vi "component orientation check.vi"(8 "error in":errorcluster, 10 "input cluster":T1, 11 "Gantry In":refnum<k24>) -> (0 "error out":errorcluster, 1 "Wrong Orientation?":bool, 2 "output cluster":T1, 3 "Gantry Out":refnum<k24>)   [LabVIEW 2021, in "Component Tray.lvclass"]
uses:
  Component Tray.lvclass
  Find Component.ctl
  Controller/Camera/Machine Vision.ctl
  C:/Program Files (x86)/Aerotech/A3200/LabVIEW/2010/Bin/Aerotech.A3200.dll
  Program Files (x86)/Aerotech/A3200/LabVIEW/2010/Bin/Aerotech.A3200.dll
  Component Tray.lvclass/Component Tray.ctl
  Controller/Motion/A3200/A3200.lvclass
  Controller/Camera/Camera.lvclass
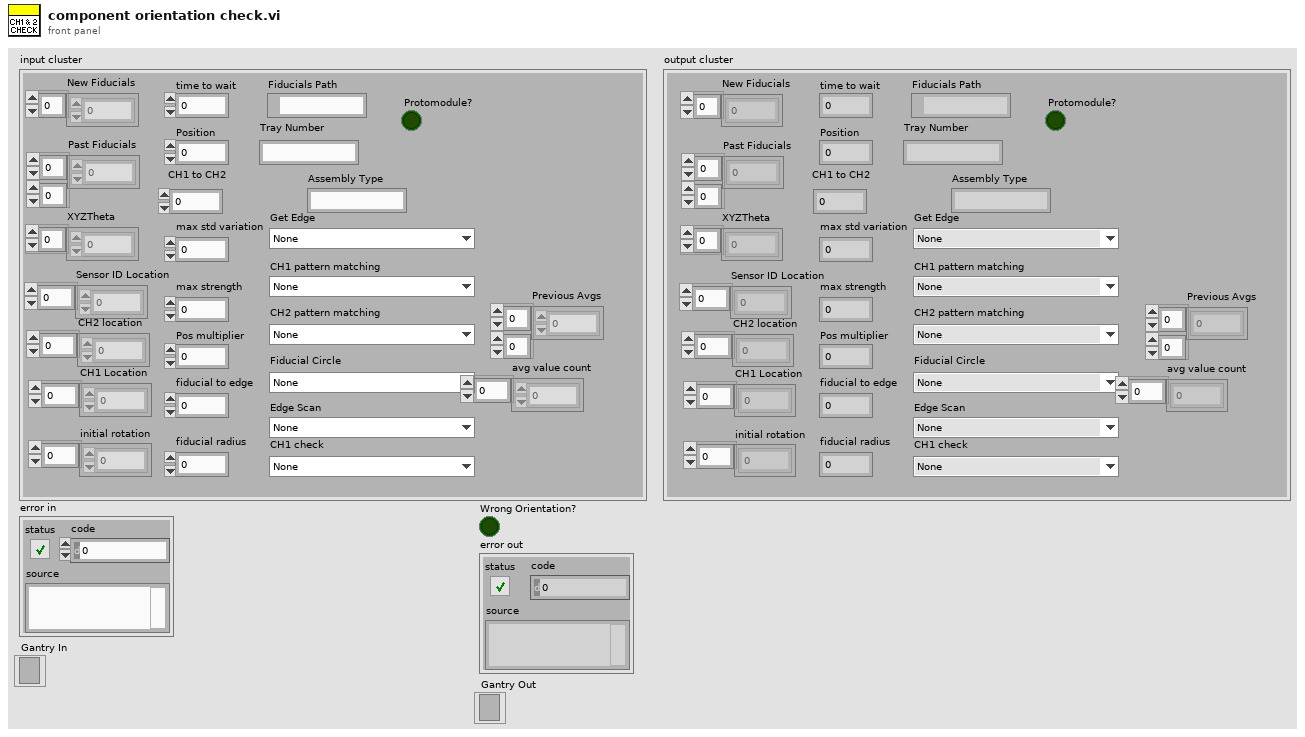
[diagram p1: front panel]
types:
  T1 = typedef "Component Tray.lvclass/Find Component.ctl" = cluster{"New Fiducials":dbl[], "Past Fiducials":dbl[][], "XYZTheta":dbl[], "Fiducials Path":path, "Position":i32, "CH1 Location":dbl[], "Sensor ID Location":dbl[], "initial rotation":dbl[], "CH2 location":dbl[], "max std variation":dbl, "max strength":dbl, "CH2 pattern matching":T2, "Fiducial Circle":T2, "Get Edge":T2, "Pos multiplier":dbl, "time to wait":u32, "fiducial to edge":dbl, "Protomodule?":bool, "Assembly Type":string, "CH1 to CH2":dbl, "Tray Number":string, "fiducial radius":dbl, "4 fiducials?":bool, "CH1 check":T2, "Edge Scan":T2, "CH1 pattern matching":T2, "Sensor Thickness":dbl, "Previous Avgs":dbl[][], "avg value count":dbl[]}
  T2 = typedef "Camera.lvclass/Machine Vision.ctl" = enum16{"None", "Assembly Tray Circle", "Assembly Tray Fiducial", "Partial Hexaboard", "sensor edge init", "HB edge init", "sensor edge pos1", "sensor edge pos2", "HB edge pos1", "HB edge pos2", "Sensor CH1-2", "HB CH1", "HB CH2", "V3 Sensor Circle", "Hexaboard Circle", "sensor CH1 check", "HB CH1 check ", "sensor ID"}
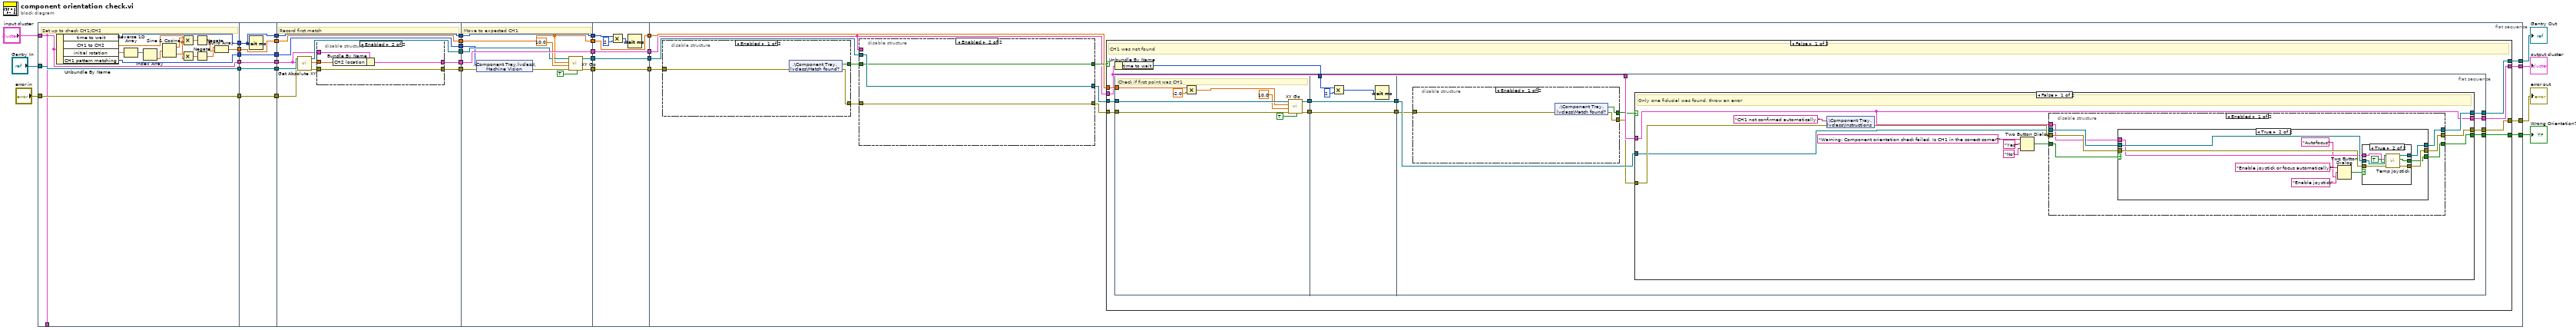
[diagram p0: block diagram]
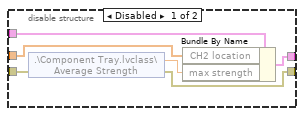
[diagram p2: hidden frame]
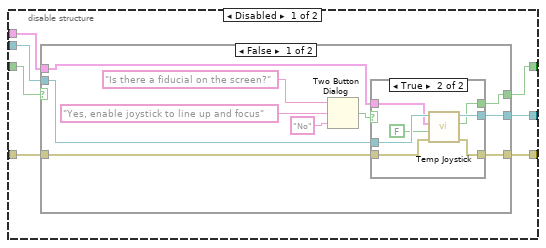
[diagram p3: hidden frame]
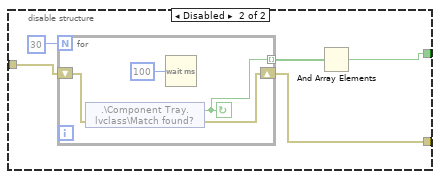
[diagram p6: hidden frame]
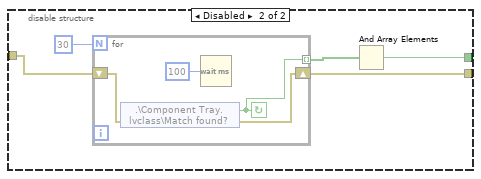
[diagram p7: hidden frame]
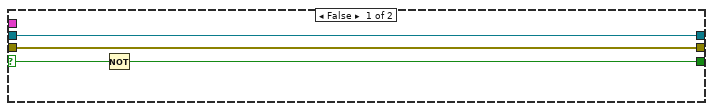
[diagram p8: hidden frame]
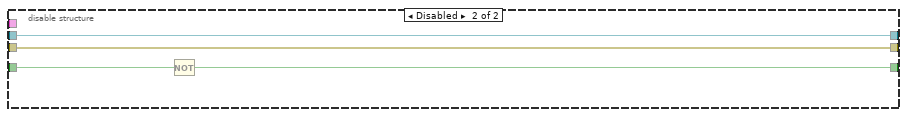
[diagram p10: hidden frame]
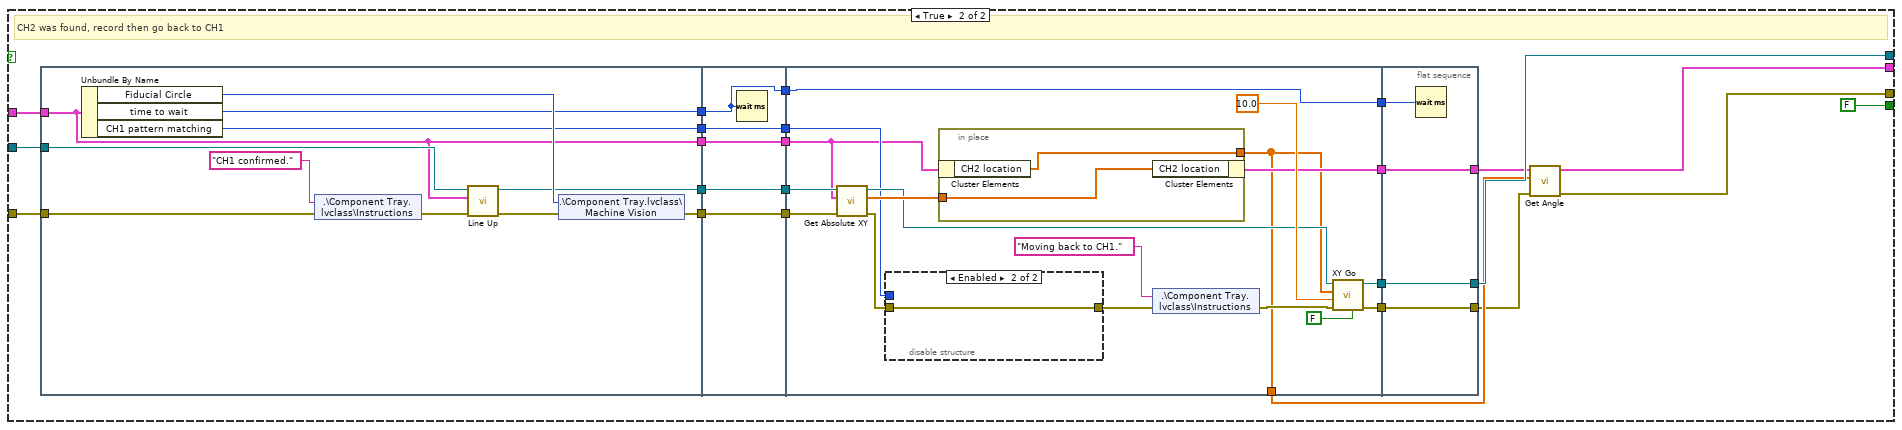
[diagram p11: hidden frame]
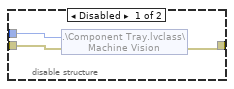
[diagram p12: hidden frame]
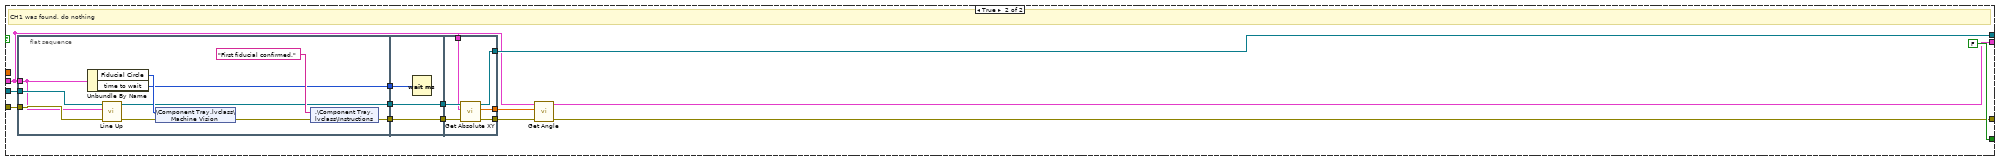
[diagram p13: hidden frame]
diagram:
  n1 = flat-sequence {
    tunnel: [w41] -> w27
    tunnel: [w40] -> w26
    tunnel: [w35] -> w25
    tunnel: [w50] -> w24
    tunnel: [w43] -> w23
    tunnel: [w42] -> w22
    tunnel: "input cluster" -> [w35]
    tunnel: "error in" -> [w40]
    tunnel: "Gantry In" -> [w41]
    tunnel: [w35] -> _
    tunnel: w27 -> [w56]
    tunnel: [w56] -> w21
    tunnel: w26 -> [w55]
    tunnel: [w55] -> w20
    tunnel: w25 -> [w54]
    tunnel: [w54] -> w19
    tunnel: w24 -> [w53]
    tunnel: [w53] -> w18
    tunnel: w23 -> [w52]
    tunnel: [w52] -> w17
    tunnel: w22 -> [w51]
    tunnel: [w51] -> w16
    tunnel: w21 -> [w66]
    tunnel: w20 -> [w65]
    tunnel: w19 -> [w57]
    tunnel: w18 -> [w60]
    tunnel: w17 -> [w63]
    tunnel: [w64] -> w15
    tunnel: [w58] -> w14
    tunnel: [w63] -> w13
    tunnel: [w62] -> w12
    tunnel: [w61] -> w11
    tunnel: w16 -> [w61]
    tunnel: [w60] -> w10
    tunnel: w15 -> [w88]
    tunnel: w14 -> [w79]
    tunnel: w13 -> [w80]
    tunnel: w12 -> [w85]
    tunnel: w11 -> [w82]
    tunnel: [w83] -> w9
    tunnel: [w84] -> w8
    tunnel: [w88] -> w7
    tunnel: w10 -> [w81]
    tunnel: [w81] -> w6
    tunnel: [w80] -> w5
    tunnel: w9 -> [w95]
    tunnel: [w95] -> w4
    tunnel: w8 -> [w94]
    tunnel: [w94] -> w3
    tunnel: w7 -> [w93]
    tunnel: [w93] -> w2
    tunnel: w6 -> [w91]
    tunnel: w5 -> [w92]
    tunnel: [w92] -> w1
    tunnel: [w105] -> w28
    tunnel: [w107] -> w29
    tunnel: [w108] -> w34
    tunnel: w4 -> [w100]
    tunnel: w3 -> [w103]
    tunnel: w2 -> [w96]
    tunnel: w1 -> [w106]
    tunnel: [w104] -> w30
    frame #0 {
      # "Set up to check CH1/CH2"
      n2 = Unbundle By Name(w35) -> ("time to wait"=w50:u32, "CH1 to CH2"=w44:dbl, "initial rotation"=w45:dbl[], "CH1 pattern matching"=w42:T2)
      n3 = Reverse 1D Array(array=w45) -> (reversed array=w46:dbl[])
      n4 = Index Array(array=w46) -> (element=w49:dbl)  [unwired: 1 in]
      n5 = Sine & Cosine(0:w49) -> (1:w48:dbl, 2:w47:dbl)
      n6 = Multiply(x=w48, y=w44) -> (x*y=w39:dbl)
      n7 = Multiply(x=w47, y=w44) -> (x*y=w37:dbl)
      n8 = Negate(x=w39) -> (-x=w38:dbl)
      n9 = Negate(x=w37) -> (-x=w36:dbl)
      n10 = Build Array(w36, w38) -> (w43:dbl[])
    }
    frame #1 {
      n11 = Wait (ms)(milliseconds to wait=w53) -> ()  [unwired: 1 out]
    }
    frame #2 {
      # "Record first match"
      n12 = call "Get Absolute XY.vi"("error in (no error)"=w65, "Component"=w57, "Gantry In"=w66) -> ("error out"=w59:errorcluster, "Abs XY"=w67:dbl[], "Gantry Out"=w62:refnum<k24>)  [unwired: 6 in]
      n13 = disable-structure shown="Enabled" {
        disable-tunnel: w57 -> [w73 w76]
        disable-tunnel: w67 -> [w72 w77]
        disable-tunnel: [w71 w75] -> w64
        disable-tunnel: w59 -> [w69 w74]
        disable-tunnel: [w68 w74] -> w58
        frame Disabled {
          n14 = shared-variable ".\\Component Tray.lvclass\\Average Strength"(error in=w69) -> (w70:dbl, error out=w68:errorcluster)
          n15 = Bundle By Name(cluster=w73, "CH2 location"=w72, "max strength"=w70) -> (w71:T1)
        }
        frame Enabled {
          n16 = Bundle By Name(cluster=w76, "CH2 location"=w77) -> (w75:T1)
        }
      }
    }
    frame #3 {
      # "Move to expected CH1"
      n17 = shared-variable ".\\Component Tray.lvclass\\Machine Vision"(w82, error in=w79) -> (error out=w78:errorcluster)
      n18 = call "XY Go.vi"("Increment?"=TRUE, "error in (no error)"=w78, "Speed"=10.0, "XY In"=w80, "Gantry In"=w85) -> ("error out"=w84:errorcluster, "Gantry Out"=w83:refnum<k24>)  [unwired: 4 in, 1 out]
    }
    frame #4 {
      n19 = Multiply(x=w91, y=u32 2) -> (x*y=w89:u32)
      n20 = Wait (ms)(milliseconds to wait=w89) -> ()  [unwired: 1 out]
    }
    frame #5 {
      n21 = disable-structure shown="Enabled" {
        disable-tunnel: [w144 w145] -> w102
        disable-tunnel: w103 -> [w143 w147]
        disable-tunnel: [w142 w146] -> w97
        frame Enabled {
          n22 = shared-variable ".\\Component Tray.lvclass\\Match found?"(error in=w143) -> (w144:bool, error out=w142:errorcluster)
        }
        frame Disabled {
          n23 = for {
            N: 30 -> [_]
            tunnel: [w150] -> w148 mode=indexing
            shift-right: [w151] -> w146
            shift-left: w147 -> [w152]
            stop <- w150 continue-if-true
            n24 = shared-variable ".\\Component Tray.lvclass\\Match found?"(error in=w152) -> (w150:bool, error out=w151:errorcluster)
            n25 = Wait (ms)(milliseconds to wait=u32 100) -> ()  [unwired: 1 out]
          }
          n26 = And Array Elements(Boolean array=w148) -> (logical AND=w145:bool)
        }
      }
      n27 = disable-structure shown="Enabled" {
        disable-tunnel: w102 -> [w115 w139]
        disable-tunnel: [w114 w139] -> w101
        disable-tunnel: w100 -> [w113 w140]
        disable-tunnel: [w112 w140] -> w99
        disable-tunnel: [w111 w141] -> w98
        disable-tunnel: w97 -> [w110 w141]
        disable-tunnel: w96 -> [w109 _]
        frame Disabled {
          n28 = case shown="False" w115 {
            selector: w115 -> [_ w138]
            tunnel: [w116 w138] -> w114
            tunnel: w113 -> [w121 w137]
            tunnel: [w120 w137] -> w112
            tunnel: [w119 w136] -> w111
            tunnel: w110 -> [w118 w136]
            tunnel: w109 -> [w117 _]
            frame False {
              n29 = Two Button Dialog(message="Is there a fiducial on the screen?", 1:"No" ("F button name (\"Cancel\")"), 2:"Yes, enable joystick to line up and focus" ("T button name (\"OK\")")) -> (T button?=w122:bool)
              n30 = case shown="True" w122 {
                selector: w122 -> [w126 _]
                tunnel: w121 -> [w128 w135]
                tunnel: [w128 w134] -> w120
                tunnel: [w127 w133] -> w119
                tunnel: w118 -> [w127 w132]
                tunnel: w117 -> [_ w130]
                tunnel: [w126 w129] -> w116
                frame False {
                }
                frame True {
                  n31 = call "Temp Joystick.vi"("error in (no error)"=w132, "Fiducial?"=FALSE ("Dialog?"), "Component"=w130, "Gantry In"=w135) -> ("error out"=w133:errorcluster, "Error?"=w129:bool, "Gantry Out"=w134:refnum<k24>)  [unwired: 5 in]
                }
              }
            }
            frame True {
            }
          }
        }
        frame Enabled {
        }
      }
      n32 = case shown="False" w101 {
        tunnel: w99 -> [w166 w327]
        tunnel: [w165 w321] -> w108
        tunnel: w98 -> [w164 w328]
        tunnel: [w163 w318] -> w107
        tunnel: w106 -> [w162 _]
        tunnel: w96 -> [w161 w317]
        tunnel: [w159 w316] -> w105
        tunnel: [w160 FALSE] -> w104
        frame False {
          # "CH1 was not found"
          n33 = Unbundle By Name(w161) -> ("time to wait"=w154:u32)
          n34 = flat-sequence {
            tunnel: w166 -> [w175]
            tunnel: w164 -> [w172]
            tunnel: w162 -> [w169]
            tunnel: [w174] -> w158
            tunnel: [w171] -> w156
            tunnel: w158 -> [w180]
            tunnel: [w180] -> w157
            tunnel: w156 -> [w179]
            tunnel: [w179] -> w155
            tunnel: w154 -> [w178]
            tunnel: [w187] -> w163
            tunnel: [w188] -> w165
            tunnel: w157 -> [w189]
            tunnel: w155 -> [w184]
            tunnel: [w181] -> w160
            tunnel: w161 -> [w186]
            tunnel: [w185] -> w159
            frame #0 {
              # "Check if first point was CH1"
              n35 = Multiply(x=w169, y=-2.0) -> (x*y=w168:dbl[])
              n36 = call "XY Go.vi"("Increment?"=TRUE, "error in (no error)"=w172, "Speed"=10.0, "XY In"=w168, "Gantry In"=w175) -> ("error out"=w171:errorcluster, "Gantry Out"=w174:refnum<k24>)  [unwired: 4 in, 1 out]
            }
            frame #1 {
              n37 = Multiply(x=w178, y=u32 2) -> (x*y=w176:u32)
              n38 = Wait (ms)(milliseconds to wait=w176) -> ()  [unwired: 1 out]
            }
            frame #2 {
              n39 = disable-structure shown="Enabled" {
                disable-tunnel: w184 -> [w192 w195]
                disable-tunnel: [w191 w194] -> w183
                disable-tunnel: [w190 w193] -> w182
                frame Enabled {
                  n40 = shared-variable ".\\Component Tray.lvclass\\Match found?"(error in=w192) -> (w190:bool, error out=w191:errorcluster)
                }
                frame Disabled {
                  n41 = for {
                    N: 30 -> [_]
                    tunnel: [w198] -> w196 mode=indexing
                    shift-right: [w199] -> w194
                    shift-left: w195 -> [w200]
                    stop <- w198 continue-if-true
                    n42 = shared-variable ".\\Component Tray.lvclass\\Match found?"(error in=w200) -> (w198:bool, error out=w199:errorcluster)
                    n43 = Wait (ms)(milliseconds to wait=u32 100) -> ()  [unwired: 1 out]
                  }
                  n44 = And Array Elements(Boolean array=w196) -> (logical AND=w193:bool)
                }
              }
              n45 = case shown="False" w182 {
                tunnel: w189 -> [w204 w272]
                tunnel: [w205 w271] -> w188
                tunnel: w183 -> [w212 w270]
                tunnel: [w211 w251] -> w187
                tunnel: w186 -> [w203 w269]
                tunnel: [w203 w249] -> w185
                tunnel: [w202 FALSE ("Error?")] -> w181
                frame False {
                  # "Only one fiducial was found, throw an error"
                  n46 = shared-variable ".\\Component Tray.lvclass\\Instructions"("CH1 not confirmed automatically." ("Instructions"), error in=w212) -> (error out=w210:errorcluster)
                  n47 = Two Button Dialog(message="Warning: Component orientation check failed. Is CH1 in the correct corner?", 1:"No" ("F button name (\"Cancel\")"), 2:"Yes" ("T button name (\"OK\")")) -> (T button?=w206:bool)
                  n48 = disable-structure shown="Enabled" {
                    disable-tunnel: [w220 w248] -> w211
                    disable-tunnel: w210 -> [w219 w248]
                    disable-tunnel: w206 -> [w218 w246]
                    disable-tunnel: [w217 w247] -> w205
                    disable-tunnel: w204 -> [w216 w247]
                    disable-tunnel: w203 -> [w215 _]
                    disable-tunnel: [w214 w245] -> w202
                    frame Enabled {
                      n49 = case shown="True" w218 {
                        selector: w218 -> [w222 _]
                        tunnel: w216 -> [w224 w234]
                        tunnel: [w224 w233] -> w217
                        tunnel: [w223 w232] -> w220
                        tunnel: w219 -> [w223 w231]
                        tunnel: w215 -> [_ w230]
                        tunnel: [w221 w229] -> w214
                        frame False {
                          n50 = Not(x=w222) -> (.not. x?=w221:bool)
                        }
                        frame True {
                          n51 = Two Button Dialog(message="Enable joystick or focus automatically?", 1:"Autofocus" ("F button name (\"Cancel\")"), 2:"Enable joystick" ("T button name (\"OK\")")) -> (T button?=w225:bool)
                          n52 = case shown="True" w225 {
                            selector: w225 -> [w235 _]
                            tunnel: w234 -> [w237 w244]
                            tunnel: [w237 w243] -> w233
                            tunnel: [w236 w242] -> w232
                            tunnel: w231 -> [w236 w241]
                            tunnel: w230 -> [_ w239]
                            tunnel: [w235 w238] -> w229
                            frame False {
                            }
                            frame True {
                              n53 = call "Temp Joystick.vi"("error in (no error)"=w241, "Fiducial?"=TRUE ("Dialog?"), "Component"=w239, "Gantry In"=w244) -> ("error out"=w242:errorcluster, "Error?"=w238:bool, "Gantry Out"=w243:refnum<k24>)  [unwired: 5 in]
                            }
                          }
                        }
                      }
                    }
                    frame Disabled {
                      n54 = Not(x=w246) -> (.not. x?=w245:bool)
                    }
                  }
                }
                frame True {
                  # "CH2 was found, record then go back to CH1"
                  n55 = flat-sequence {
                    tunnel: w269 -> [w273]
                    tunnel: [w276] -> w264
                    tunnel: [w282] -> w262
                    tunnel: [w280] -> w260
                    tunnel: [w273] -> w258
                    tunnel: [w281] -> w256
                    tunnel: w270 -> [w278]
                    tunnel: w272 -> [w277]
                    tunnel: w264 -> [w288]
                    tunnel: [w288] -> w263
                    tunnel: w262 -> [w287]
                    tunnel: [w287] -> w261
                    tunnel: w260 -> [w286]
                    tunnel: [w286] -> w259
                    tunnel: w258 -> [w285]
                    tunnel: [w285] -> w257
                    tunnel: w256 -> [w284]
                    tunnel: [w284] -> w255
                    tunnel: [w298] -> w268
                    tunnel: [w299] -> w267
                    tunnel: [w300] -> w266
                    tunnel: [w305] -> w265
                    tunnel: w255 -> [w297]
                    tunnel: w257 -> [w289]
                    tunnel: w259 -> [w294]
                    tunnel: w261 -> [w305]
                    tunnel: w263 -> [w295]
                    tunnel: [w290] -> w253
                    tunnel: [w313] -> w250
                    tunnel: [w314] -> w252
                    tunnel: [w315] -> w271
                    tunnel: w268 -> [w315]
                    tunnel: w267 -> [w314]
                    tunnel: w266 -> [w313]
                    tunnel: w265 -> [w312]
                    frame #0 {
                      n56 = Unbundle By Name(w273) -> ("Fiducial Circle"=w283:T2, "time to wait"=w282:u32, "CH1 pattern matching"=w281:T2)
                      n57 = shared-variable ".\\Component Tray.lvclass\\Instructions"("CH1 confirmed." ("Instructions"), error in=w278) -> (error out=w274:errorcluster)
                      n58 = call "Line Up.vi"("error IO"=w274, "Component"=w273, "Gantry In"=w277) -> ("error out"=w275:errorcluster, "Gantry Out"=w276:refnum<k24>)  [unwired: 6 in, 1 out]
                      n59 = shared-variable ".\\Component Tray.lvclass\\Machine Vision"(w283, error in=w275) -> (error out=w280:errorcluster)
                    }
                    frame #1 {
                      n60 = Wait (ms)(milliseconds to wait=w287) -> ()  [unwired: 1 out]
                    }
                    frame #2 {
                      n61 = call "Get Absolute XY.vi"("error in (no error)"=w294, "Component"=w289, "Gantry In"=w295) -> ("error out"=w296:errorcluster, "Abs XY"=w304:dbl[], "Gantry Out"=w301:refnum<k24>)  [unwired: 6 in]
                      n62 = disable-structure shown="Enabled" {
                        disable-tunnel: w297 -> [w308 _]
                        disable-tunnel: w296 -> [w307 w309]
                        disable-tunnel: [w306 w309] -> w292
                        frame Disabled {
                          n63 = shared-variable ".\\Component Tray.lvclass\\Machine Vision"(w308, error in=w307) -> (error out=w306:errorcluster)
                        }
                        frame Enabled {
                        }
                      }
                      n64 = in-place {
                        in-place-border: w304 -> [w311]
                        in-place-border: [w310] -> w290
                        n65 = in-place-cluster #1(w289) -> ("CH2 location"=w310:dbl[])
                        n66 = in-place-cluster #1("CH2 location"=w311) -> (w300:T1)
                      }
                      n67 = shared-variable ".\\Component Tray.lvclass\\Instructions"("Moving back to CH1." ("Instructions"), error in=w292) -> (error out=w291:errorcluster)
                      n68 = call "XY Go.vi"("Increment?"=FALSE, "error in (no error)"=w291, "Speed"=10.0, "XY In"=w290, "Gantry In"=w301) -> ("error out"=w299:errorcluster, "Gantry Out"=w298:refnum<k24>)  [unwired: 4 in, 1 out]
                    }
                    frame #3 {
                      n69 = Wait (ms)(milliseconds to wait=w312) -> ()  [unwired: 1 out]
                    }
                  }
                  n70 = call "Get Angle.vi"("error in"=w252, "array"=w253, "input cluster"=w250) -> ("error out"=w251:errorcluster, "output cluster"=w249:T1)  [unwired: 7 in]
                }
              }
            }
          }
        }
        frame True {
          # "CH1 was found, do nothing"
          n71 = flat-sequence {
            tunnel: w328 -> [w337]
            tunnel: w327 -> [w335]
            tunnel: w317 -> [w330]
            tunnel: [w334] -> w326
            tunnel: [w332] -> w325
            tunnel: [w331] -> w324
            tunnel: w326 -> [w342]
            tunnel: w325 -> [w341]
            tunnel: w324 -> [w340]
            tunnel: [w342] -> w323
            tunnel: [w341] -> w322
            tunnel: w323 -> [w347]
            tunnel: w322 -> [w348]
            tunnel: w317 -> [w343]
            tunnel: [w346] -> w319
            tunnel: [w345] -> w320
            tunnel: [w344] -> w321
            frame #0 {
              n72 = Unbundle By Name(w330) -> ("Fiducial Circle"=w339:T2, "time to wait"=w331:u32)
              n73 = call "Line Up.vi"("error IO"=w337, "Component"=w330, "Gantry In"=w335) -> ("error out"=w336:errorcluster, "Gantry Out"=w334:refnum<k24>)  [unwired: 6 in, 1 out]
              n74 = shared-variable ".\\Component Tray.lvclass\\Machine Vision"(w339, error in=w336) -> (error out=w333:errorcluster)
              n75 = shared-variable ".\\Component Tray.lvclass\\Instructions"("First fiducial confirmed." ("Instructions"), error in=w333) -> (error out=w332:errorcluster)
            }
            frame #1 {
              n76 = Wait (ms)(milliseconds to wait=w340) -> ()  [unwired: 1 out]
            }
            frame #2 {
              n77 = call "Get Absolute XY.vi"("error in (no error)"=w348, "Component"=w343, "Gantry In"=w347) -> ("error out"=w346:errorcluster, "Abs XY"=w345:dbl[], "Gantry Out"=w344:refnum<k24>)  [unwired: 6 in]
            }
          }
          n78 = call "Get Angle.vi"("error in"=w319, "array"=w320, "input cluster"=w317) -> ("error out"=w318:errorcluster, "output cluster"=w316:T1)  [unwired: 7 in]
        }
      }
    }
  }
  "Wrong Orientation?" <- w30
  "output cluster" <- w28
  "error out" <- w29
  "Gantry Out" <- w34
